vi "Shutdown.vi"(8 "error in":errorcluster, 11 "Modbus slave in":refnum<class "Modbus Slave.lvclass">) -> (0 "error out":errorcluster)   [LabVIEW 2012, in "Modbus Slave.lvclass"]
doc: "Performs any actions needed to shutdown and clean up the Modbus instance provided. For a slave instance, this will force a shutdown of the slave daemon and close all connections to the physical bus."
uses:
  Modbus Slave.lvclass
  Modbus Slave.lvclass/Modbus Slave.ctl
  Network Protocol/Network Slave/Network Slave.lvclass
  Data Model/Device Data Model.lvclass
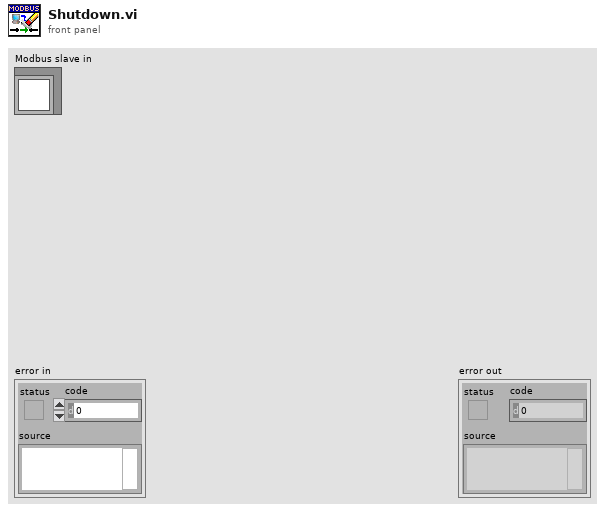
[diagram p1: front panel]
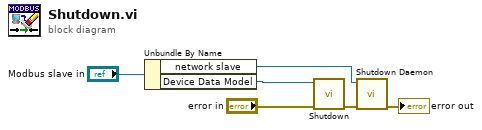
[diagram p0: block diagram]
diagram:
  n1 = Unbundle By Name("Modbus slave in") -> ("network slave"=w3:refnum<class "Network Slave.lvclass">, "Device Data Model"=w1:refnum<class "Device Data Model.lvclass">)
  n2 = call-dynamic "Shutdown.vi"("error in"="error in", "device data model in"=w1) -> ("error out"=w4:errorcluster)  [unwired: 9 in]
  n3 = call-dynamic "Shutdown Daemon.vi"("error in"=w4, "network slave in"=w3) -> ("error out"=→"error out":errorcluster)  [unwired: 9 in]
